vi "Exercise4.5-FM_RTL-SDR_RX - FIR.vi"() -> ()   [LabVIEW 2013]
uses:
  <vilib>/sound2/lvsound2.llb/Sound Data Format.ctl
  <vilib>/sound2/lvsound2.llb/Sound Output Write (DBL Single).vi
  <instrlib>/rtlsdr/rtlsdr.lvlib
panel:
  out "Constellation":cdb[](graph)
  out "Waveform Chart":u32(graph)=133
  out "Time elapse (ms)":u32
  in  "Device index":u32
  out "Samples Acquired":u32
  out "DevRefnum":u64
  out "error out":errorcluster
  in  "sound format":T1={"sample rate (S/s)"=44100.0, "number of channels"=1, "bits per sample"=16}
  in  "stop":bool
  in  "Center frequency":u32=92700000
  in  "IQ rate":u32=286650
  out "error out":errorcluster
  # "FM Receiver"
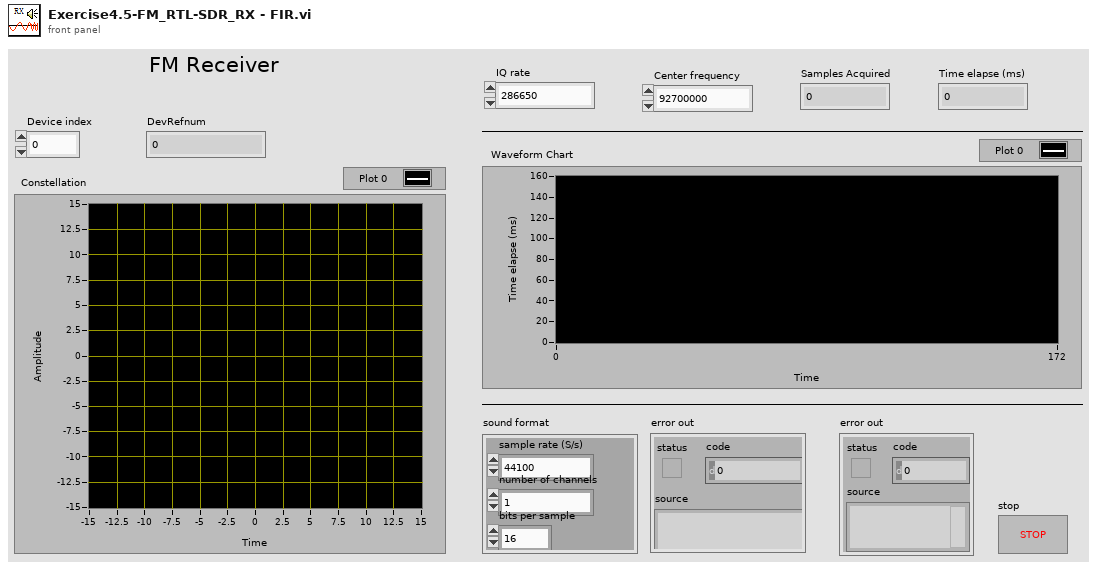
[diagram p1: front panel]
types:
  T1 = typedef "Sound Data Format.ctl" = cluster{"sample rate (S/s)":dbl, "number of channels":i32, "bits per sample":i32}
  T2 = typedef "Sound Output Task ID.ctl" = u32
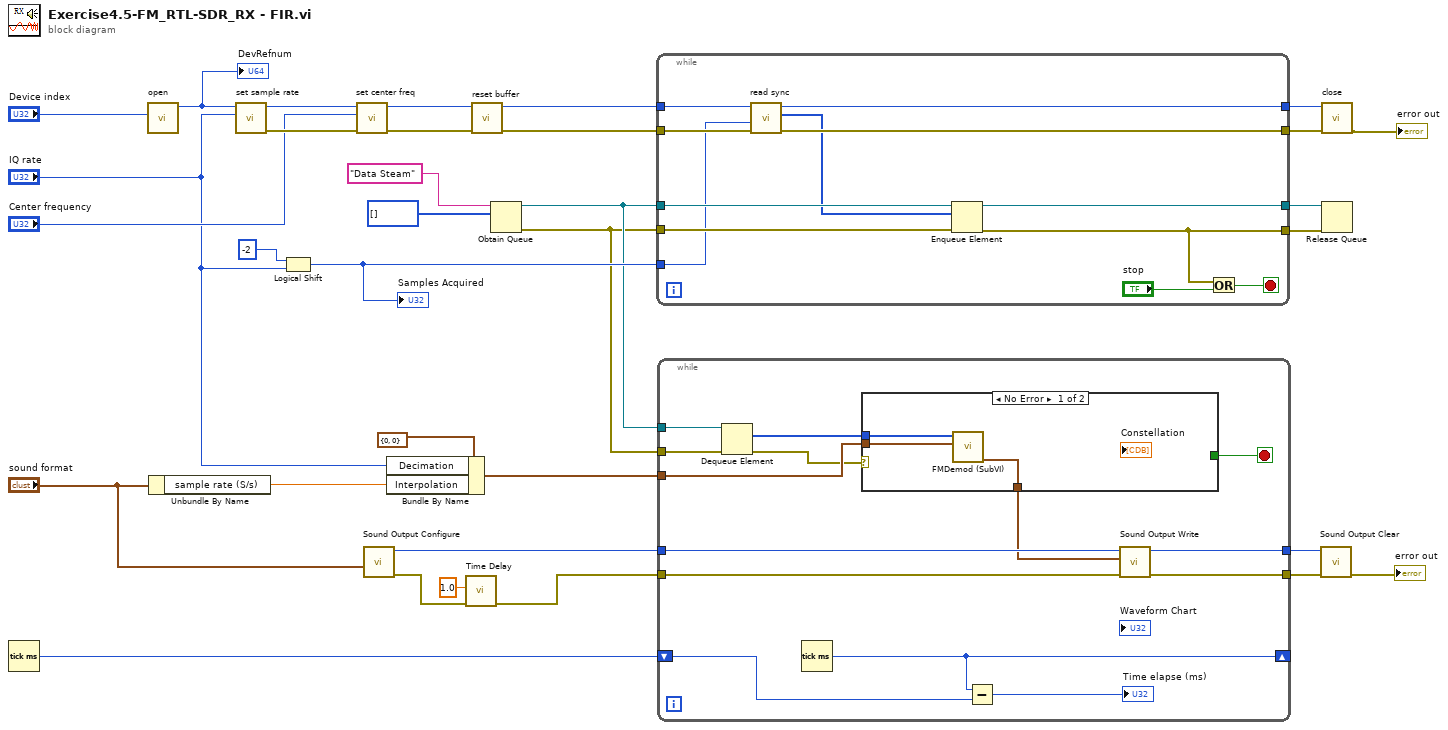
[diagram p0: block diagram]
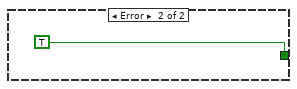
[diagram p2: hidden frame]
diagram:
  n1 = Tick Count (ms)() -> (millisecond timer value=w1:u32)
  n2 = call <instrlib>:"open.vi"("index"="Device index") -> ("DevRefnum"=w26:u64)  [unwired: 9 in, 1 out]
  "DevRefnum" <- w26
  n3 = Unbundle By Name("sound format") -> ("sample rate (S/s)"=w18:dbl)
  n4 = call <instrlib>:"set sample rate.vi"("rate"="IQ rate", "DevRefnum"=w26) -> ("error out"=w28:errorcluster, "DevRefnum"=w30:u64)  [unwired: 7 in, 1 out]
  n5 = Logical Shift(y=i16 -2, x="IQ rate") -> (x << y=w8:u32)
  "Samples Acquired" <- w8
  n6 = call <instrlib>:"set center freq.vi"("error in (no error)"=w28, "freq"="Center frequency", "DevRefnum"=w30) -> ("error out"=w27:errorcluster, "DevRefnum"=w29:u64)  [unwired: 6 in, 1 out]
  n7 = call <vilib>:"Sound Output Configure.vi"("sound format"="sound format") -> ("error out"=w12:errorcluster, "task ID"=w5:T2)  [unwired: 9 in]
  n8 = Bundle By Name(cluster=cluster{"Interpolation":i32, "Decimation":i32} {"Interpolation"=0, "Decimation"=0}, "Decimation"="IQ rate", "Interpolation"=w18) -> (w13:cluster{"Interpolation":i32, "Decimation":i32})
  n9 = call "Time Delay"("error in (no error)"=w12, "Delay Time (s)"=1.0) -> ("error out"=w4:errorcluster)  [unwired: 9 in]
  n10 = call <instrlib>:"reset buffer.vi"("error in (no error)"=w27, "DevRefnum"=w29) -> ("error out"=w23:errorcluster, "DevRefnum"=w24:u64)  [unwired: 8 in]
  n11 = Obtain Queue(name (unnamed)="Data Steam", element data type=u8[] [] ("buf 2")) -> (queue out=w3:refnum<queue>, error out=w2:errorcluster)  [unwired: 3 in, 1 out]
  n12 = while {
    tunnel: [w43] -> w21
    tunnel: w24 -> [w45]
    tunnel: w23 -> [w44]
    tunnel: [w42] -> w20
    tunnel: w8 -> [w36]
    tunnel: w3 -> [w41]
    tunnel: [w40] -> w16
    tunnel: w2 -> [w39]
    tunnel: [w34] -> w15
    stop <- w37 stop-if-true
    n13 = call <instrlib>:"read sync.vi"("error in (no error)"=w44, "len"=w36, "DevRefnum"=w45) -> ("error out"=w42:errorcluster, "buf 2"=w35:u8[], "DevRefnum"=w43:u64)  [unwired: 6 in]
    n14 = Enqueue Element(queue=w41, element=w35, error in (no error)=w39) -> (queue out=w40:refnum<queue>, error out=w34:errorcluster)  [unwired: 1 in, 1 out]
    n15 = Or(x=w34, y="stop") -> (x .or. y?=w37:bool)
  }
  n16 = while {
    tunnel: w3 -> [w59]
    tunnel: w13 -> [w56]
    tunnel: w2 -> [w57]
    tunnel: [w54] -> w7
    tunnel: [w53] -> w6
    tunnel: w5 -> [w52]
    tunnel: w4 -> [w49]
    shift-right: [w48] -> _
    shift-left: w1 -> [w47]
    stop <- w55 stop-if-true
    n17 = Dequeue Element(queue=w59, error in (no error)=w57) -> (element=w58:u8[], error out=w51:errorcluster)  [unwired: 1 in, 2 out]
    n18 = Tick Count (ms)() -> (millisecond timer value=w48:u32)
    n19 = case shown="No Error" w51 {
      tunnel: w58 -> [w62 _]
      tunnel: [w60 _] -> w50
      tunnel: w56 -> [w61 _]
      tunnel: [_ TRUE] -> w55
      frame No Error {
        n20 = call "FMDemod (SubVI).vi"("Cluster"=w61, "buf in"=w62) -> ("Waveform"=w60:waveform(dbl))  [unwired: 8 in, 1 out]
      }
      frame Error {
      }
    }
    n21 = Subtract(x=w48, y=w47) -> (x-y=→"Time elapse (ms)":u32)
    n22 = call-poly <vilib>:"Sound Output Write.vi"("error in (no error)"=w49, "data"=w50, "task ID"=w52) -> ("error out"=w53:errorcluster, "task ID out"=w54:T2)  [unwired: 7 in]
  }
  n23 = call <vilib>:"Sound Output Clear.vi"("error in (no error)"=w6, "task ID"=w7) -> ("error out"=→"error out":errorcluster)  [unwired: 9 in]
  n24 = call <instrlib>:"close.vi"("error in (no error)"=w20, "DevRefnum"=w21) -> ("error out"=→"error out":errorcluster)  [unwired: 8 in, 1 out]
  n25 = Release Queue(queue=w16, error in (no error)=w15) -> ()  [unwired: 1 in, 3 out]
